vi "control6acater.vi"() -> ()   [LabVIEW 2018]
uses:
  <vilib>/eio/EIONode/EIONode.xnode
  <vilib>/rvi/eio/common/nirviEmuTemplateMethod_errors.vi
panel:
  in  "Array":i16[](array[numeric])
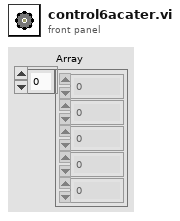
[diagram p1: front panel]
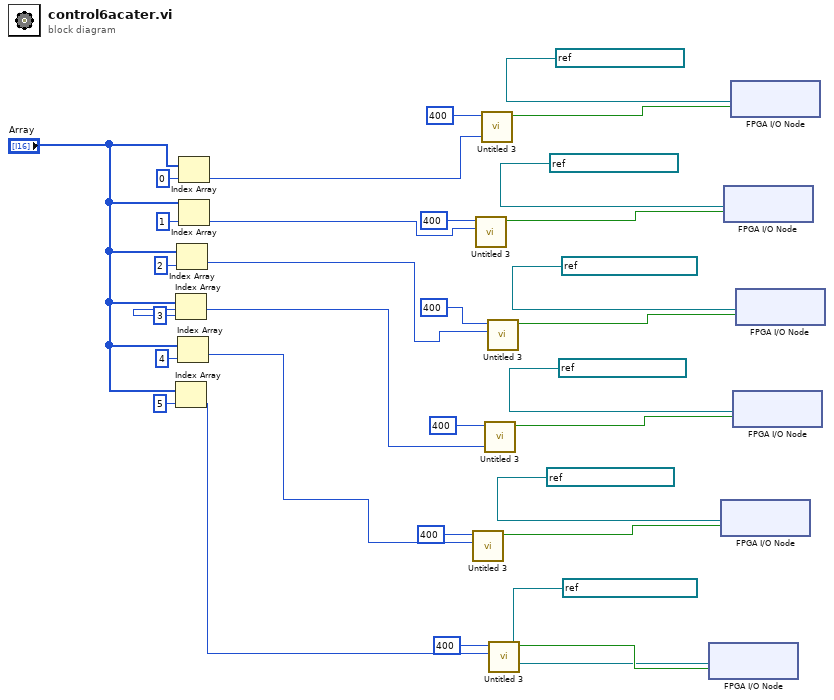
[diagram p0: block diagram]
diagram:
  n1 = Index Array(array="Array", index=3) -> (element=w4:i16)
  n2 = Index Array(array="Array", index=5) -> (element=w2:i16)
  n3 = Index Array(array="Array", index=2) -> (element=w5:i16)
  n4 = Index Array(array="Array", index=4) -> (element=w3:i16)
  n5 = Index Array(array="Array", index=0) -> (element=w22:i16)
  n6 = Index Array(array="Array", index=1) -> (element=w6:i16)
  n7 = call "Untitled 3.vi"("Duty Cycle"=w3, "Period (Ticks)"=u32 400) -> ("PWM Out"=w12:bool)  [unwired: 8 in, 1 out]
  n8 = call "Untitled 3.vi"("Duty Cycle"=w6, "Period (Ticks)"=u32 400) -> ("PWM Out"=w21:bool)  [unwired: 8 in, 1 out]
  n9 = call "Untitled 3.vi"("Duty Cycle"=w22, "Period (Ticks)"=u32 400) -> ("PWM Out"=w1:bool)  [unwired: 8 in, 1 out]
  n10 = call "Untitled 3.vi"("Duty Cycle"=w4, "Period (Ticks)"=u32 400) -> ("PWM Out"=w15:bool)  [unwired: 8 in, 1 out]
  n11 = call "Untitled 3.vi"("Duty Cycle"=w5, "Period (Ticks)"=u32 400) -> ("PWM Out"=w18:bool)  [unwired: 8 in, 1 out]
  n12 = call "Untitled 3.vi"("Duty Cycle"=w2, "Period (Ticks)"=u32 400) -> ("PWM Out"=w9:bool)  [unwired: 8 in, 1 out]
  n13 = xnode "FPGA I/O Node"("I/O Item"=w9, "FPGA I/O In"=refnum<k21> "ConnectorB/DIO10") -> ()  [unwired: 1 out]
  n14 = xnode "FPGA I/O Node"("I/O Item"=w12, "FPGA I/O In"=refnum<k21> "ConnectorB/DIO9") -> ()  [unwired: 1 out]
  n15 = xnode "FPGA I/O Node"("I/O Item"=w21, "FPGA I/O In"=refnum<k21> "ConnectorA/DIO9") -> ()  [unwired: 1 out]
  n16 = xnode "FPGA I/O Node"("I/O Item"=w1, "FPGA I/O In"=refnum<k21> "ConnectorA/DIO8") -> ()  [unwired: 1 out]
  n17 = xnode "FPGA I/O Node"("I/O Item"=w15, "FPGA I/O In"=refnum<k21> "ConnectorB/DIO8") -> ()  [unwired: 1 out]
  n18 = xnode "FPGA I/O Node"("I/O Item"=w18, "FPGA I/O In"=refnum<k21> "ConnectorA/DIO10") -> ()  [unwired: 1 out]
